vi "Get Channel Actual Values.vi"(8 "error in (no error)":errorcluster, 9 "System Time":dbl[](array[numeric]), 10 "Column Data":T1, 11 "TDMS in":refnum<k34>) -> (0 "error out":errorcluster, 2 "Actual Values":dbl[](array[numeric]), 3 "TDMS Out":refnum<k34>)   [LabVIEW 2011]
uses:
  Controls/Test Column Data.ctl
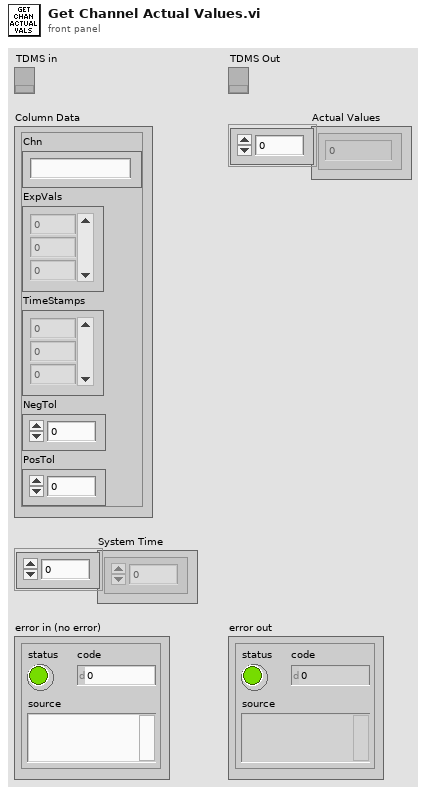
[diagram p1: front panel]
types:
  T1 = typedef "Test Column Data.ctl" = cluster{"Chn":string, "ExpVals":dbl[], "TimeStamps":i64[], "NegTol":dbl, "PosTol":dbl}
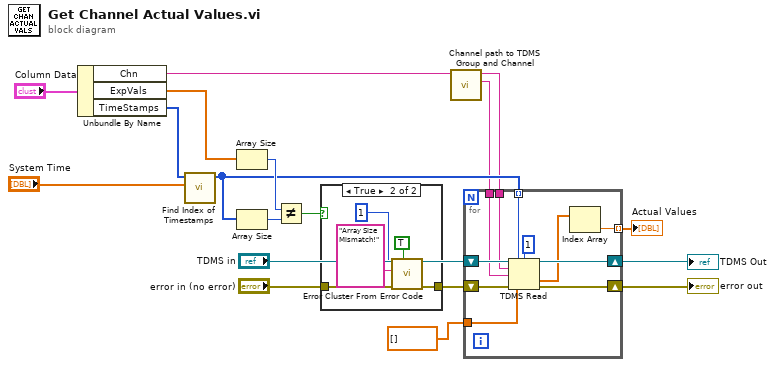
[diagram p0: block diagram]
diagram:
  n1 = Unbundle By Name("Column Data") -> ("Chn"=w6:string, "ExpVals"=w15:dbl[], "TimeStamps"=w9:i64[])
  n2 = call "Find Index of Timestamps.vi"("System Time (s)"="System Time", "Test TimeStamps (us)"=w9) -> ("Test TDMS Offsets"=w10:i64[])  [unwired: 9 in]
  n3 = Array Size(array=w15) -> (size(s)=w12:i32)
  n4 = Array Size(array=w10) -> (size(s)=w11:i32)
  n5 = Not Equal?(x=w12, y=w11) -> (x != y?=w14:bool)
  n6 = case shown="True" w14 {
    tunnel: [w19 w24] -> w13
    tunnel: "error in (no error)" -> [w19 w23]
    frame False {
    }
    frame True {
      n7 = call <vilib>:"Error Cluster From Error Code.vi"("show call chain? (False)"=TRUE, "error in (no error)"=w23, "error message (\"\")"="Array Size Mismatch!" ("error message (\"\")"), "error code (0)"=1) -> ("error out"=w24:errorcluster)  [unwired: 5 in]
    }
  }
  n8 = call "Channel path to TDMS Group and Channel.vi"("Channel Path"=w6) -> ("TDMS Channel"=w7:string, "TDMS Group"=w8:string)  [unwired: 9 in]
  n9 = for {
    tunnel: w7 -> [w33]
    tunnel: w8 -> [w32]
    shift-right: [w31] -> w4
    shift-left: w13 -> [w35]
    tunnel: w10 -> [w30] mode=indexing
    tunnel: dbl[] [] -> [w28]
    shift-right: [w27] -> w5
    shift-left: "TDMS in" -> [w34]
    tunnel: [w25] -> w17 mode=indexing
    n10 = TDMS Read(0:w34, 1:w30, 2:i64 1 ("count (-1: all)"), 5:w32, 7:w33, 11:w35, 12:w28) -> (4:w27:refnum<k34>, 10:w26:dbl[], 15:w31:errorcluster)  [unwired: 1 in, 3 out]
    n11 = Index Array(array=w26) -> (element=w25:dbl)  [unwired: 1 in]
  }
  "Actual Values" <- w17
  "TDMS Out" <- w5
  "error out" <- w4
